vi "Commit To Database.vi"(8 "error in (no error)":errorcluster, 10 "TableName(\"\")":string, 11 "ExcuseNotesHandler in":refnum<class "ExcuseNotesHandler.lvclass">) -> (0 "error out":errorcluster, 3 "ExcuseNotesHandler out":refnum<class "ExcuseNotesHandler.lvclass">)   [LabVIEW 2015, in "ExcuseNotesHandler.lvclass"]
uses:
  ExcuseNotesHandler.lvclass
  ExcuseNotesHandler.lvclass/ExcuseNotesHandler.ctl
  API/_Database/Database.lvclass
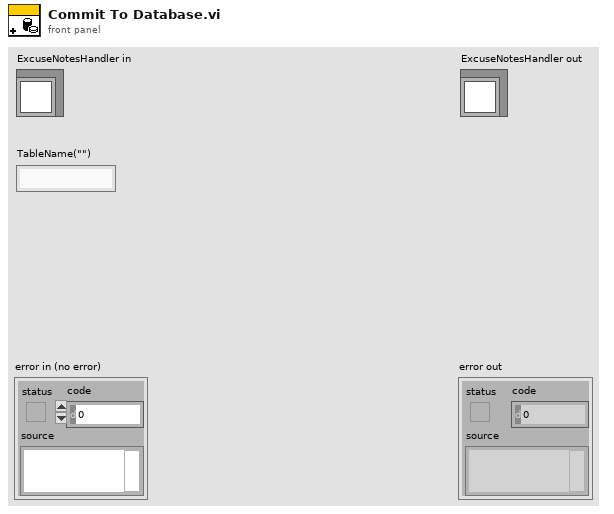
[diagram p1: front panel]
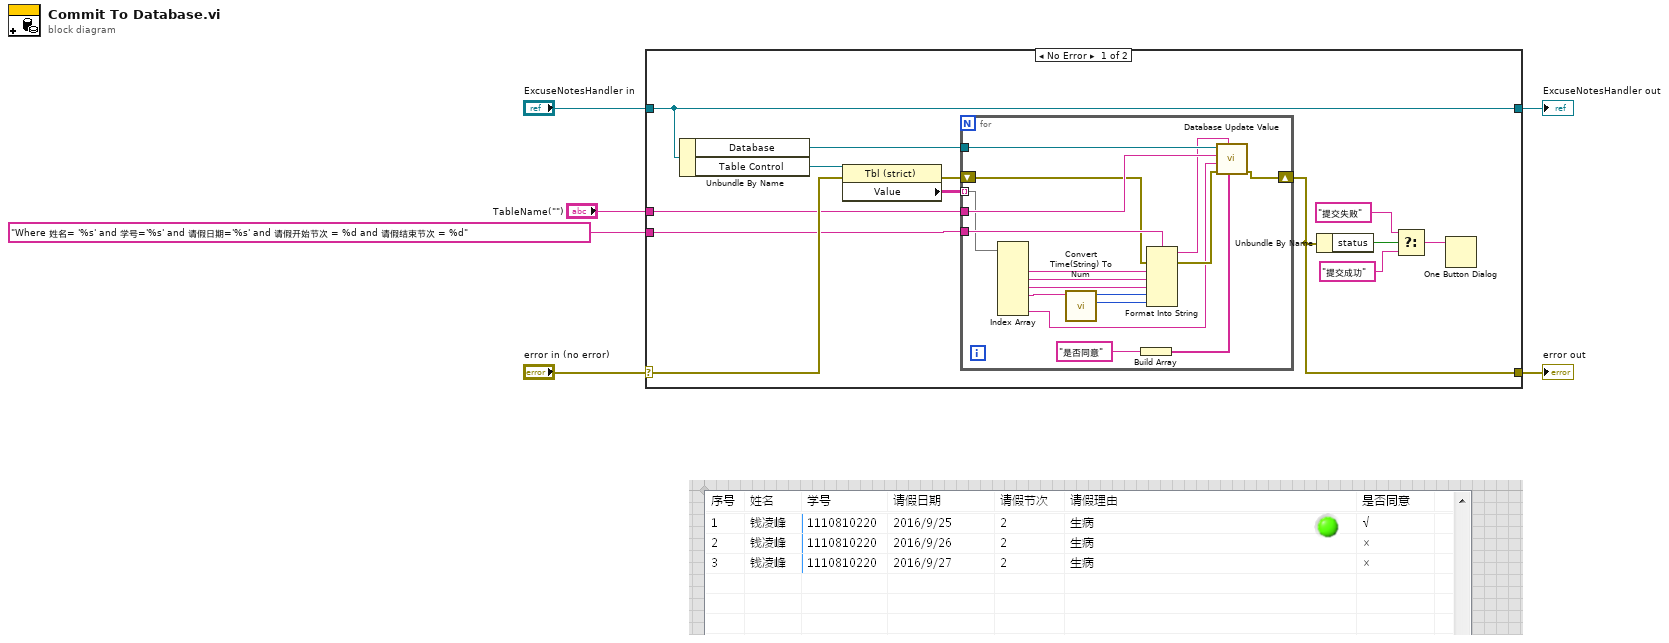
[diagram p0: block diagram]
diagram:
  n1 = case shown="No Error" "error in (no error)" {
    selector: "error in (no error)" -> [w17 w38]
    tunnel: [w7 w38] -> w5
    tunnel: [w19 w37] -> w3
    tunnel: "ExcuseNotesHandler in" -> [w19 w37]
    tunnel: "TableName(\"\")" -> [w13 _]
    tunnel: "Where 姓名= '%s' and 学号='%s' and 请假日期='%s' and 请假开始节次 = %d and 请假结束节次 = %d" ("condition") -> [w12 _]
    frame No Error {
      n2 = Unbundle By Name(w19) -> ("Database"=w14:refnum<class "Database.lvclass">, "Table Control"=w18:refnum<vi>)
      n3 = property class="Tbl (strict)"(reference=w18, error in=w17) -> (error out=w15:errorcluster, "Value"=w16:string[][])  [unwired: 1 out]
      n4 = for {
        tunnel: w16 -> [w29] mode=indexing
        tunnel: w14 -> [w36]
        tunnel: w13 -> [w35]
        tunnel: w12 -> [w34]
        shift-right: [w30] -> w7
        shift-left: w15 -> [w32]
        n5 = Index Array(array=w29) -> (element #2=w28:string, element #3=w27:string, element #4=w26:string, element #5=w25:string, element #7=w20:string)  [unwired: 7 in, 2 out]
        n6 = call "Convert Time(String) To Num.vi"("ExcuseTime(\"\")"=w25) -> ("Time2"=w23:i32, "Time1"=w24:i32)  [unwired: 9 in]
        n7 = Build Array("是否同意") -> (w21:string[])
        n8 = Format Into String(format string=w34, error in=w32, w28, w27, w26, w24, w23) -> (resulting string=w33:string, error out=w31:errorcluster)  [unwired: 1 in]
        n9 = call "Database Update Value.vi"("columns"=w21, "condition"=w33, "error in (no error)"=w31, "data"=w20, "table"=w35, "Database in"=w36) -> ("error out"=w30:errorcluster)  [unwired: 4 in, 1 out]
      }
      n10 = Unbundle By Name(w7) -> ("status"=w11:bool)
      n11 = Select(t="提交失败", s=w11, f="提交成功") -> (s? t:f=w8:string)
      n12 = One Button Dialog(message=w8) -> ()  [unwired: 1 in, 1 out]
    }
    frame Error {
    }
  }
  "error out" <- w5
  "ExcuseNotesHandler out" <- w3
